vi "VoltageOut Setter.vi"(0 "DeviceReference":T1, 3 "Update Frequency (Hz)":dbl=100.0, 5 "Output":dbl, 7 "EnableFOC":bool=TRUE) -> (4 "DeviceReference Out":T1)   [LabVIEW 2020]
doc: "Request a specified voltage.\nThis control mode will attempt to apply the specified voltage to the motor. If the supply voltage is below the requested voltage, the motor controller will output the supply voltage."
uses:
  DeviceReference.ctl
  <userlib>/CTRE_PhoenixTools/CTRE_PhoenixTools.lvlib
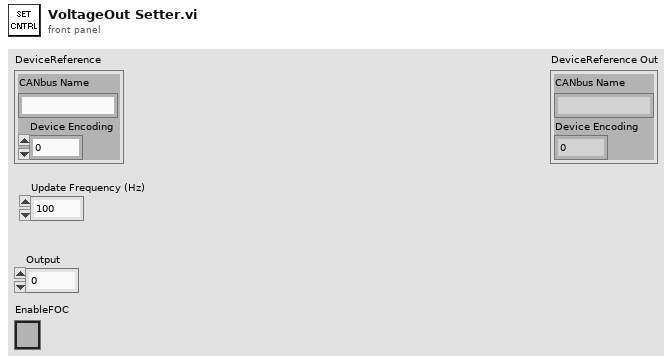
[diagram p1: front panel]
types:
  T1 = typedef "DeviceReference.ctl" = cluster{"CANbus Name":string, "Device Encoding":u32}
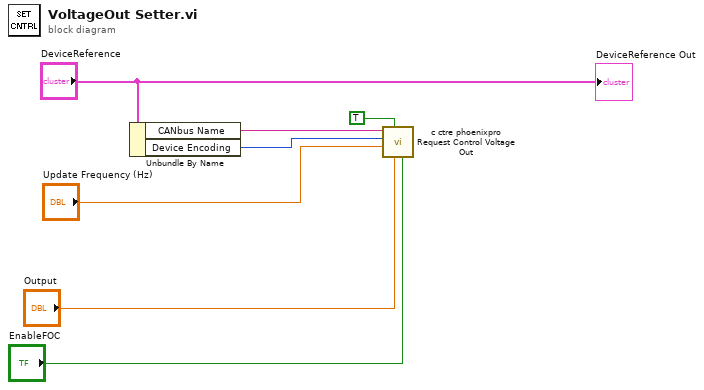
[diagram p0: block diagram]
diagram:
  n1 = Unbundle By Name("DeviceReference") -> ("CANbus Name"=w6:string, "Device Encoding"=w5:u32)
  n2 = call <userlib>:"c ctre phoenixpro Request Control Voltage Out.vi"("EnableFOC"="EnableFOC", "Output"="Output", "cancelOtherRequests"=TRUE, "updateTime"="Update Frequency (Hz)", "ecuEncoding"=w5, "canbus"=w6) -> ()  [unwired: 4 in, 2 out]
  "DeviceReference Out" <- "DeviceReference"
